vi "Butterfly_PullDown RC2_ERMod.vi"(0 "Semiconductor Module Context":T1, 1 "RFPins":string[](array[string]), 2 "current level":dbl=0.01 format="%_6p", 3 "R Thresholds":dbl[](array[numeric]), 5 "error in (no error)":errorcluster, 6 "PD_Pin":string="SMU_PD", 7 "Start_v":dbl=10.0 format="%#_13g", 9 "Stop_v":dbl=41.0 format="%#_13g", 11 "Step_v":dbl=1.0) -> (14 "Semiconductor Module Context Out":T1, 19 "error out":errorcluster)   [LabVIEW 2013]
uses:
  <vilib>/NI_TestStand_SemiconductorModule/NI_TestStand_Semiconductor_Module.lvlibp/PinMap/General/SemiconductorModuleContext.ctl
  <instrlib>/niDCPower/nidcpower.llb/niDCPower Wait For Event - Event.ctl
  <vilib>/NI_TestStand_SemiconductorModule/NI_TestStand_Semiconductor_Module.lvlibp/PinMap/DC Power/PinToNIDCPowerSession.vi
  <vilib>/NI_TestStand_SemiconductorModule/NI_TestStand_Semiconductor_Module.lvlibp/PinMap/DC Power/PinsToNIDCPowerSessions.vi
  <vilib>/NI_TestStand_SemiconductorModule/NI_TestStand_Semiconductor_Module.lvlibp/PinMap/General/Publish/PublishDataDoubleFunctionalTest.vi
  <vilib>/NI_TestStand_SemiconductorModule/NI_TestStand_Semiconductor_Module.lvlibp
panel:
  out "Full R Array":dbl[][][](array[numeric])
  out "step":i32
  out "Instrument Session":refnum<k15>
  out "sites and pins loop iter":i32
  out "Channel List":string
  out "BF values":dbl[](array[numeric])
  out "BF Names":string[](array[string])
  out "R Array":dbl[](array[numeric])
  out "BFSamples":i32
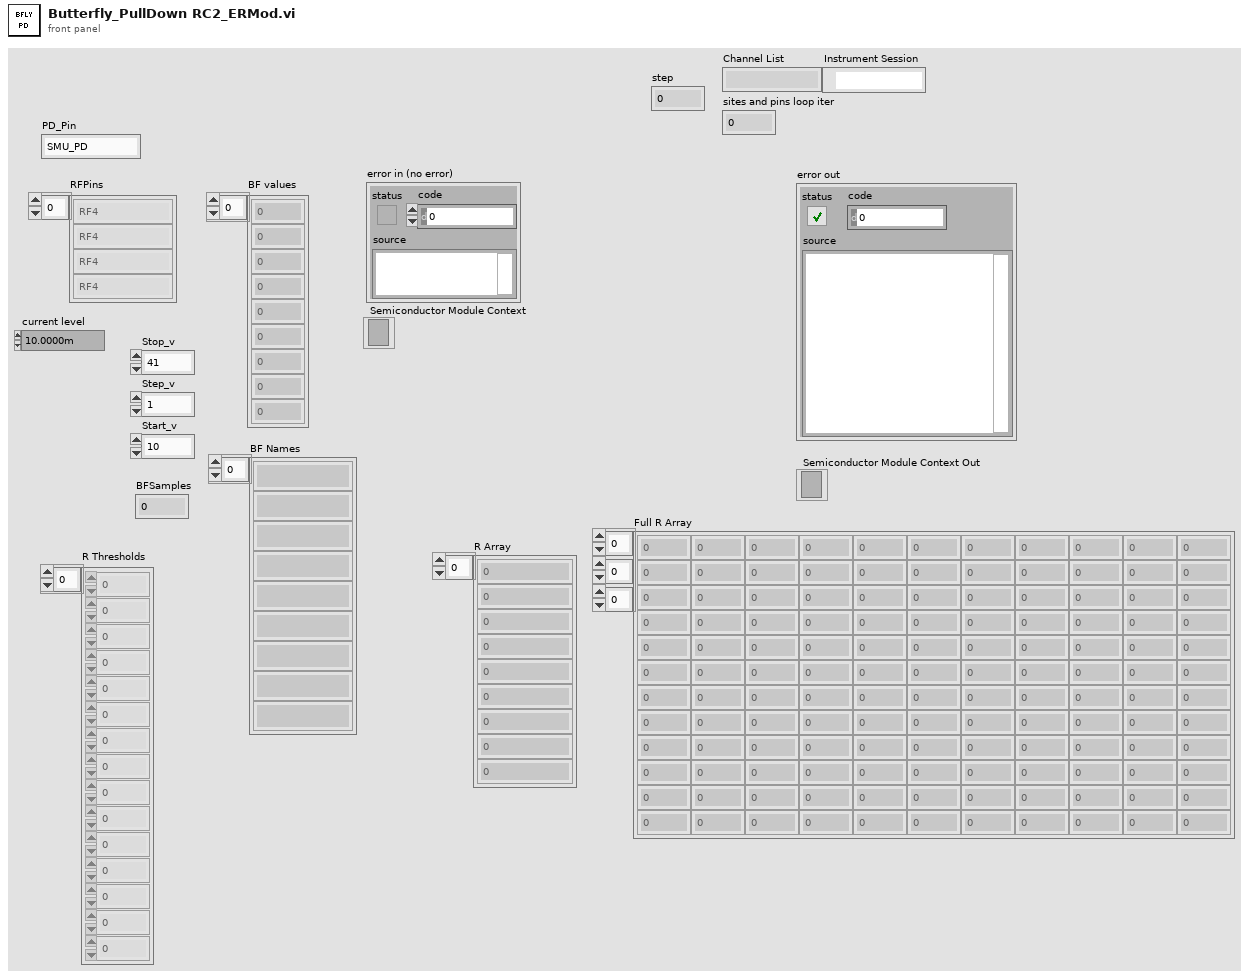
[diagram p1: front panel]
types:
  T1 = typedef "NI_TestStand_Semiconductor_Module.lvlibp/SemiconductorModuleContext.ctl" = refnum<k7>
  T2 = typedef "niDCPower Wait For Event - Event.ctl" = i32
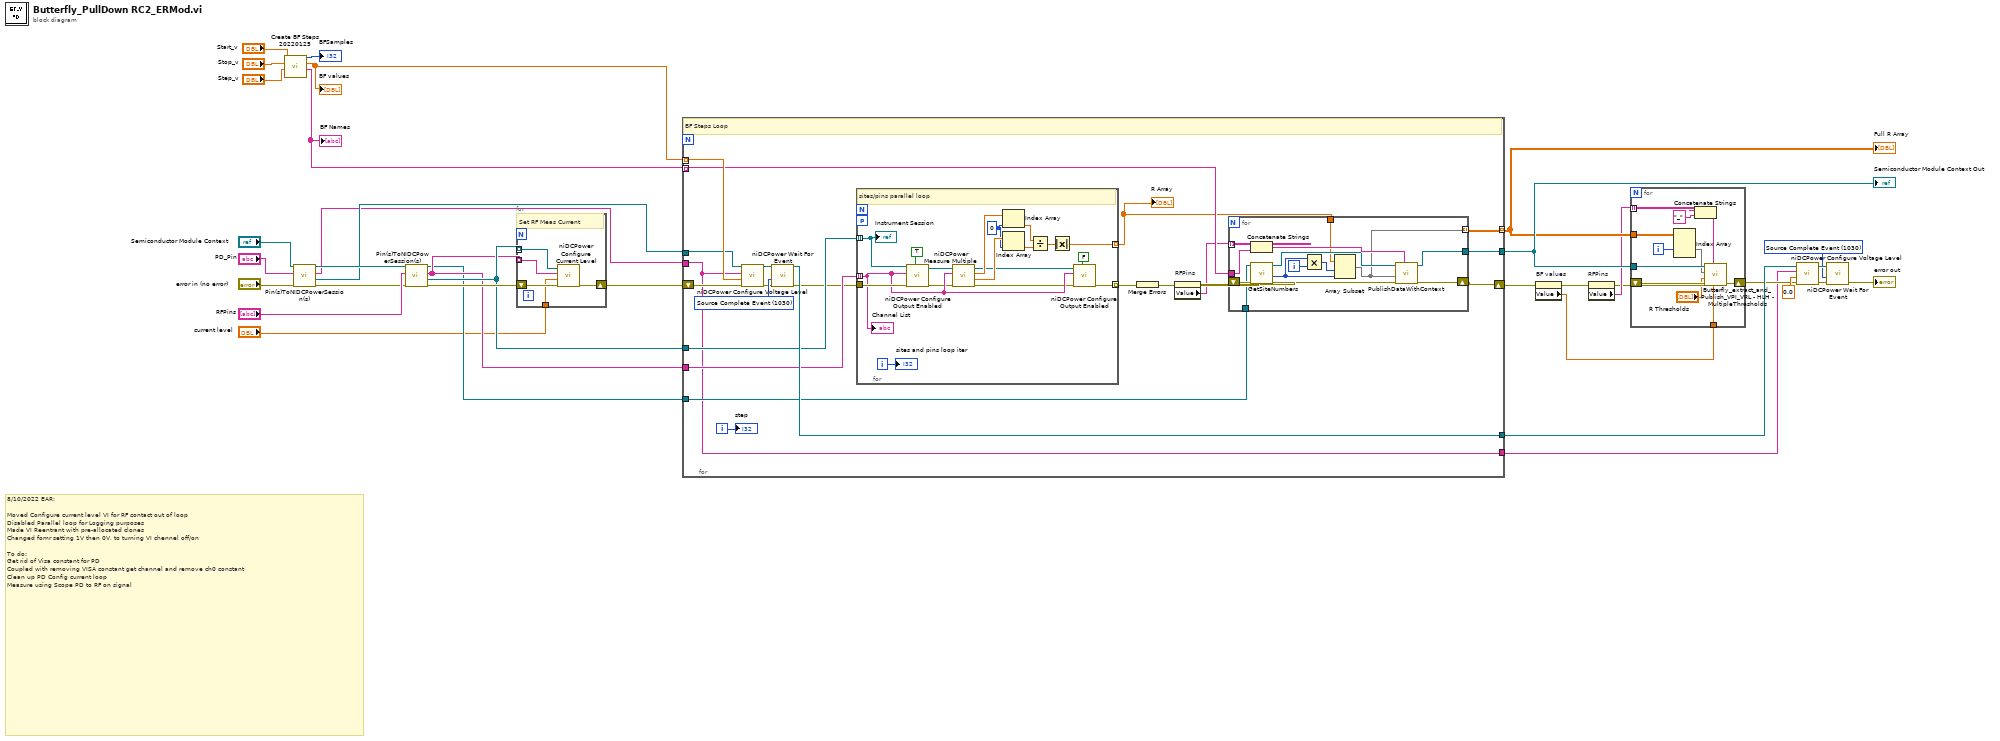
[diagram p0: block diagram]
diagram:
  w26 = T2 1030 items=["Source Complete Event"=1030, "Measure Complete Event"=1031, "Sequence Iteration Complete Event"=1032, "Sequence Engine Done Event"=1033, "Pulse Complete Event"=1051, "Ready For Pulse Trigger Event"=1052] ("event")
  # "8/10/2022 EAR:\n\nMoved Configure current level VI for RF contact out of loop\nDisabled Parallel loop for Logging purposes\nMade VI Reentrant with pre-allocated clones\nChanged fomr setting 1V then 0V, to turning VI chennel off/on\n\nTo do:\nGet rid of Visa constant for PD\nCoupled with removing VISA constant get channel and remove ch0 constant\nClean up PD Config current loop\nMeasure using Scope PD to RF on signal"
  n1 = call "Create BF Steps 20220125.vi"("Step_v"="Step_v", "Stop_v"="Stop_v", "Start_v"="Start_v") -> ("BF Names"=w25:string[], "BF values"=w24:dbl[], "BFSamples"=→"BFSamples":i32)  [unwired: 6 in]
  "BF Names" <- w25
  "BF values" <- w24
  n2 = call-poly <vilib>:"Pin(s)ToNIDCPowerSession(s).vi"("error in (no error)"="error in (no error)", "Pin"="PD_Pin", "Semiconductor Module Context"="Semiconductor Module Context") -> ("error out"=w12:errorcluster, "Instrument Session"=w9:refnum<k15>, "Channel List"=w8:string, "Semiconductor Module Context Out"=w13:T1)  [unwired: 4 in, 1 out]
  n3 = call-poly <vilib>:"Pin(s)ToNIDCPowerSession(s).vi"("error in (no error)"=w12, "Pins"="RFPins", "Semiconductor Module Context"=w13) -> ("error out"=w21:errorcluster, "Instrument Sessions"=w19:refnum<k15>[], "Channel Lists"=w18:string[], "Semiconductor Module Context Out"=w16:T1)  [unwired: 4 in, 1 out]
  n4 = for {
    shift-right: [w39] -> w20
    shift-left: w21 -> [w40]
    tunnel: w19 -> [w38] mode=indexing
    tunnel: w18 -> [w37] mode=indexing
    tunnel: "current level" -> [w36]
    # "Set RF Meas Current"
    n5 = call <instrlib>:"niDCPower Configure Current Level.vi"("error in (no error)"=w40, "current level"=w36, "channel name"=w37, "instrument handle"=w38) -> ("error out"=w39:errorcluster)  [unwired: 6 in, 1 out]
  }
  n6 = for {
    shift-right: [w41] -> w3
    shift-left: w20 -> [w59]
    tunnel: w24 -> [w58] mode=indexing
    tunnel: w9 -> [w57]
    tunnel: [w56] -> w30
    tunnel: w25 -> [w54] mode=indexing
    tunnel: [w53] -> w22
    tunnel: w19 -> [w52]
    tunnel: w18 -> [w51]
    tunnel: w16 -> [w48]
    tunnel: [w47] -> w15 mode=indexing
    tunnel: w8 -> [w42]
    tunnel: [w42] -> w5
    i -> [w55]
    w61 = T2 1030 items=["Source Complete Event"=1030, "Measure Complete Event"=1031, "Sequence Iteration Complete Event"=1032, "Sequence Engine Done Event"=1033, "Pulse Complete Event"=1051, "Ready For Pulse Trigger Event"=1052] ("event")
    # "BF Steps Loop"
    n7 = call <instrlib>:"niDCPower Configure Voltage Level.vi"("error in (no error)"=w59, "voltage level"=w58, "channel name"=w42, "instrument handle"=w57) -> ("error out"=w60:errorcluster, "instrument handle out"=w62:refnum<k15>)  [unwired: 6 in]
    n8 = call <instrlib>:"niDCPower Wait For Event.vi"("error in (no error)"=w60, "event"=w61, "instrument handle"=w62) -> ("error out"=w50:errorcluster, "instrument handle out"=w56:refnum<k15>)  [unwired: 7 in]
    n9 = for {
      workers-P: _ -> [_]
      tunnel: w52 -> [w88] mode=indexing
      tunnel: w51 -> [w85] mode=indexing
      tunnel: [w87] -> w49 mode=indexing
      tunnel: w50 -> [w89]
      tunnel: [w86] -> w46 mode=indexing
      i -> [w94]
      w77 = 0 ("index")
      # "sites/pins parallel loop"
      n10 = call <instrlib>:"niDCPower Configure Output Enabled.vi"("error in (no error)"=w89, "output enabled"=TRUE, "channel name"=w85, "instrument handle"=w88) -> ("error out"=w81:errorcluster, "instrument handle out"=w80:refnum<k15>)  [unwired: 6 in]
      n11 = call <instrlib>:"niDCPower Measure Multiple.vi"("error in (no error)"=w81, "channel name"=w85, "instrument handle"=w80) -> ("error out"=w78:errorcluster, "current measurements"=w84:dbl[], "voltage measurements"=w93:dbl[], "instrument handle out"=w79:refnum<k15>)  [unwired: 5 in]
      n12 = Index Array(array=w93, index=w77) -> (element=w91:dbl)
      n13 = Index Array(array=w84, index=w77) -> (element=w92:dbl)
      n14 = Divide(x=w91, y=w92) -> (x/y=w90:dbl)
      n15 = Absolute Value(x=w90) -> (abs(x)=w87:dbl)
      n16 = call <instrlib>:"niDCPower Configure Output Enabled.vi"("error in (no error)"=w78, "output enabled"=FALSE, "channel name"=w85, "instrument handle"=w79) -> ("error out"=w86:errorcluster)  [unwired: 6 in, 1 out]
      "Channel List" <- w85
      "sites and pins loop iter" <- w94
      "Instrument Session" <- w88
    }
    "R Array" <- w49
    n17 = Merge Errors(w46) -> (w45:errorcluster)
    n18 = property on="RFPins" class="Arr (strict)"(error in=w45) -> (error out=w44:errorcluster, "Value"=w43:string[])  [unwired: 1 in, 1 out]
    n19 = for {
      tunnel: w43 -> [w75] mode=indexing
      tunnel: w54 -> [w74]
      tunnel: [w70] -> w53
      tunnel: w49 -> [w65]
      tunnel: w48 -> [w64]
      tunnel: [w63] -> w47 mode=indexing
      shift-right: [w72] -> w41
      shift-left: w44 -> [w66]
      i -> [w76]
      n20 = Concatenate Strings(w75, w74) -> (w71:string)
      n21 = call <vilib>:"GetSiteNumbers.vi"("error in (no error)"=w66, "Semiconductor Module Context"=w64) -> ("error out"=w69:errorcluster, "Number Of Sites"=w67:i32, "Semiconductor Module Context Out"=w68:T1)  [unwired: 6 in, 1 out]
      n22 = Multiply(x=w67, y=w76) -> (x*y=w73:i32)
      n23 = Array Subset(array=w65, index=w73, length=w67) -> (w63:dbl[])
      n24 = call-poly <vilib>:"PublishDataWithContext.vi"("Published Data Id"=w71, "error in (no error)"=w69, "Data In"=w63, "Semiconductor Module Context"=w68) -> ("error out"=w72:errorcluster, "Semiconductor Module Context Out"=w70:T1)  [unwired: 6 in]
    }
    "step" <- w55
  }
  "Semiconductor Module Context Out" <- w22
  "Full R Array" <- w15
  n25 = property on="BF values" class="Arr (strict)"(error in=w3) -> (error out=w2:errorcluster, "Value"=w1:dbl[])  [unwired: 1 in, 1 out]
  n26 = property on="RFPins" class="Arr (strict)"(error in=w2) -> (error out=w6:errorcluster, "Value"=w7:string[])  [unwired: 1 in, 1 out]
  n27 = for {
    tunnel: w7 -> [w101] mode=indexing
    shift-right: [w102] -> w23
    shift-left: w6 -> [w103]
    tunnel: w22 -> [w98]
    tunnel: w15 -> [w97]
    tunnel: w1 -> [w95]
    i -> [w105]
    n28 = Index Array(array=w97, index (dim 1)=w105) -> (element=w96:dbl[][])  [unwired: 2 in]
    n29 = Concatenate Strings(w101, "_" ("string")) -> (w99:string)
    n30 = call "Butterfly_extract_and_Publish_VPI_VRL - HLH - MultipleThresholds.vi"("Voltages Array"=w95, "ID Prefix"=w99, "error in (no error)"=w103, "Thresholds"="R Thresholds", "Result Array In"=w96, "Semiconductor Module Context"=w98) -> ("error out"=w102:errorcluster)  [unwired: 5 in]
  }
  n31 = call <instrlib>:"niDCPower Configure Voltage Level.vi"("error in (no error)"=w23, "voltage level"=0.0, "channel name"=w5, "instrument handle"=w30) -> ("error out"=w29:errorcluster, "instrument handle out"=w27:refnum<k15>)  [unwired: 6 in]
  n32 = call <instrlib>:"niDCPower Wait For Event.vi"("error in (no error)"=w29, "event"=w26, "instrument handle"=w27) -> ("error out"=→"error out":errorcluster)  [unwired: 7 in, 1 out]
